vi "ReservationMemory.vi"(2 "Width":i32, 3 "Height":i32, 5 "Error IN LabVIEW":errorcluster) -> (18 "Error OUT Toolkit":i32, 19 "Error OUT LabVIEW":errorcluster)   [LabVIEW 2018]
doc: "It reserves in GPU memory two spaces for 1D Arrays U8 to perform operations inside it. It receives the width and height that the image should have, previously transformed into an array.\n\nIt is the initial VI of the DLL, this should pass the variable error to \"CopyDataToGPU\"."
uses:
  dll/LibreriaAutis_3.dll
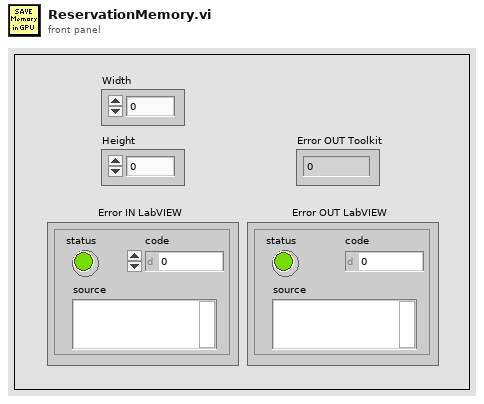
[diagram p1: front panel]
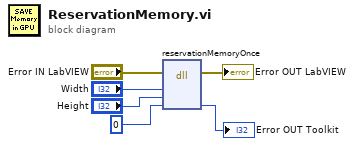
[diagram p0: block diagram]
diagram:
  n1 = dll-call lib="C:/Users/AUTIS/Desktop/LibreriaAUTIS/LabVIEW/dll/LibreriaAutis_3.dll" fn="reservationMemoryOnce"(error in="Error IN LabVIEW", "w"="Width", "h"="Height", "error"=0) -> (error out=→"Error OUT LabVIEW":errorcluster, "error"=→"Error OUT Toolkit":i32)  [unwired: 5 in, 1 out]
